vi "SaveToFileSettings.vi"(8 "ErrorIn":errorcluster) -> (0 "ErrorOut":errorcluster)   [LabVIEW 2019]
uses:
  FilePathToSaveAction.ctl
panel:
  in  "Close":bool
  in  "Index":u32
  in  "FilesNames":string="pomiar"
  in  "DirPath":path
  # "Wybierz ścieżkę do folderu na dane pomiarowe:"
  # "Podaj nazwę dla nowego zestawu plików z danymi:"
  # "Podaj nr indeksu plików, od którego rozpocznie się numeracja.\nUwaga! Jeśli istnieje już plik z daną nazwą i podanym numerem indeksu,\nistniejący plik zostanie nadpisany."
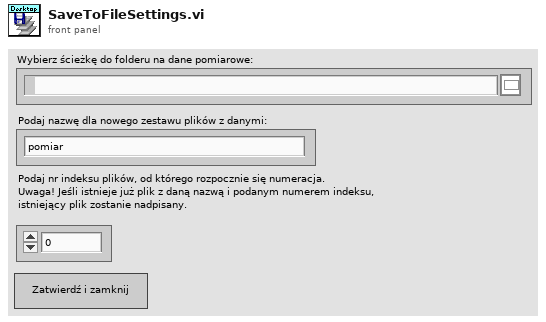
[diagram p1: front panel]
types:
  T1 = typedef "FilePathToSaveAction.ctl" = enum16{"Build new path", "Update index", "Get file path", "Get current settings"}
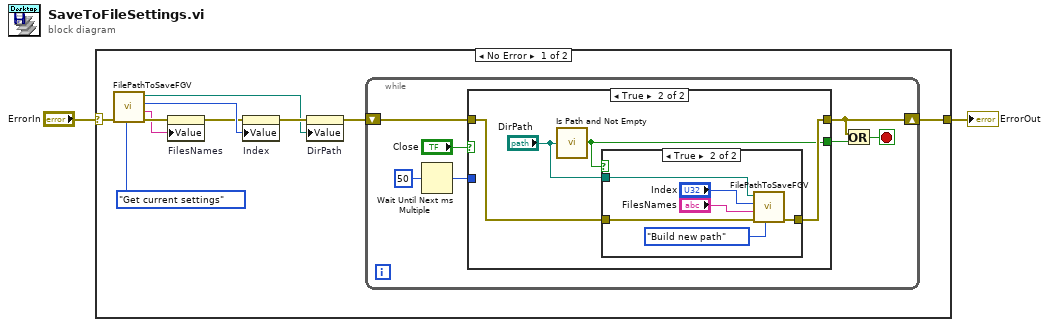
[diagram p0: block diagram]
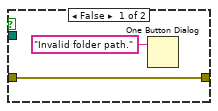
[diagram p3: hidden frame]
diagram:
  n1 = case shown="No Error" "ErrorIn" {
    selector: "ErrorIn" -> [w11 w33]
    tunnel: [w12 w33] -> w2
    frame No Error {
      n2 = call "FilePathToSaveFGV.vi"("FilePathToSaveAction"=FilePathToSaveAction."Get current settings", "ErrorIn"=w11) -> ("ErrorOut"=w8:errorcluster, "FileNamesOut"=w7:string, "IndexOut"=w9:u32, "File path"=w3:path)  [unwired: 6 in]
      n3 = property on="FilesNames" class="Str"(error in=w8, "Value"=w7) -> (error out=w6:errorcluster)  [unwired: 1 in, 1 out]
      n4 = property on="Index" class="DigNum (strict)"(error in=w6, "Value"=w9) -> (error out=w5:errorcluster)  [unwired: 1 in, 1 out]
      n5 = property on="DirPath" class="Path"(error in=w5, "Value"=w3) -> (error out=w4:errorcluster)  [unwired: 1 in, 1 out]
      n6 = while {
        shift-right: [w13] -> w12
        shift-left: w4 -> [w18]
        stop <- w14 stop-if-true
        n7 = Wait Until Next ms Multiple(millisecond multiple=u32 50) -> (millisecond timer value=w17:u32)
        n8 = case shown="True" "Close" {
          tunnel: w18 -> [w20 w24]
          tunnel: w17 -> [_ _]
          tunnel: [w20 w23] -> w13
          tunnel: [_ w22] -> w15
          frame False {
          }
          frame True {
            n9 = call <vilib>:"Is Path and Not Empty.vi"("path"="DirPath") -> ("Is Path and Not Empty?"=w22:bool)  [unwired: 4 in]
            n10 = case shown="True" w22 {
              tunnel: w24 -> [w26 w30]
              tunnel: [w26 w29] -> w23
              tunnel: "DirPath" -> [_ w27]
              frame False {
                n11 = One Button Dialog(message="Invalid folder path.") -> ()  [unwired: 1 in, 1 out]
              }
              frame True {
                n12 = call "FilePathToSaveFGV.vi"("FilePathToSaveAction"=FilePathToSaveAction."Build new path", "ErrorIn"=w30, "FilesNames"="FilesNames", "Index"="Index", "DirPath"=w27) -> ("ErrorOut"=w29:errorcluster)  [unwired: 3 in, 3 out]
              }
            }
          }
        }
        n13 = Or(x=w13, y=w15) -> (x .or. y?=w14:bool)
      }
    }
    frame Error {
    }
  }
  "ErrorOut" <- w2
